vi "casestructure.vi"() -> ()   [LabVIEW 2015]
panel:
  in  "stop":bool
  in  "Combo Box":string(combo)
  in  "Ring":u16(ring) items=["DIVISION", "ADD", "SUB", "MULTIPLY"]
  in  "Choice":string
  in  "Choice":i32
  out "result":dbl
  in  "op 2":dbl
  in  "op1":dbl
  # "CALCULATOR"
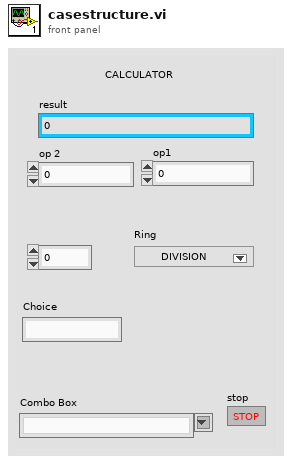
[diagram p1: front panel]
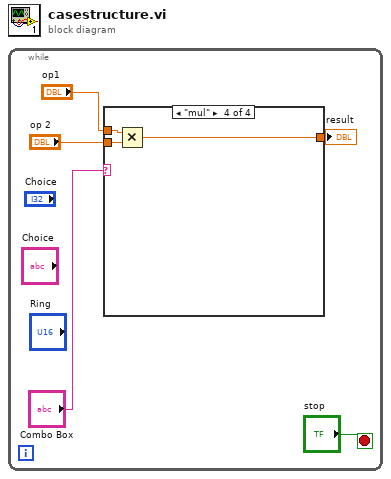
[diagram p0: block diagram]
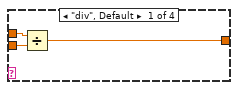
[diagram p2: hidden frame]
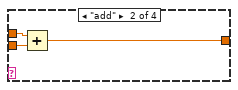
[diagram p3: hidden frame]
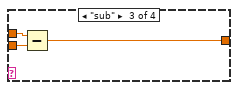
[diagram p4: hidden frame]
diagram:
  n1 = while {
    stop <- "stop" stop-if-true
    n2 = case shown="\"mul\"" "Combo Box" {
      tunnel: "op1" -> [w8 w11 w12 w17]
      tunnel: "op 2" -> [w6 w10 w13 w16]
      tunnel: [w7 w9 w14 w15] -> w3
      frame "div", Default {
        n3 = Divide(x=w8, y=w6) -> (x/y=w7:dbl)
      }
      frame "add" {
        n4 = Add(x=w11, y=w10) -> (x+y=w9:dbl)
      }
      frame "sub" {
        n5 = Subtract(x=w12, y=w13) -> (x-y=w14:dbl)
      }
      frame "mul" {
        n6 = Multiply(x=w17, y=w16) -> (x*y=w15:dbl)
      }
    }
    "result" <- w3
  }
